vi "Fourier_Maple_Test.vi"() -> ()   [LabVIEW 2013]
uses:
  Hello Optotune Lens (30.06.2014)/Calibration.ctl
  <vilib>/Instr/_visa.llb/VISA Configure Serial Port (Instr).vi
panel:
  in  "f2k":dbl(slide)=114.95741056218058 min=80.0 max=200.0 scale=80.0..200.0
  in  "f1k":dbl(slide)=192.02725724020442 min=80.0 max=200.0 scale=80.0..200.0
  in  "Fourier/Abbildung":bool
  in  "f1i":dbl(slide)=80.0 min=80.0 max=200.0 step=5.0 scale=80.0..200.0
  in  "f2i":dbl(slide)=100.64735945485519 min=80.0 max=200.0 scale=80.0..200.0
  out "error out 2":errorcluster
  in  "error in (no error) 2":errorcluster
  in  "VISA resource name 2":string="COM14"
  out "I_min":dbl
  out "I_max":dbl
  in  "Calibration":T1={"Max Current A"=293.0, "Max Current B"=293.0, "UCL A"=300.0, "UCL B"=300.0, "LCL A"=0.0, "LCL B"=0.0} {"Max Current A" format="%#_g mA"; "Max Current B" format="%#_g mA"; "UCL A" format="%#_g mA"; "LCL A" format="%#_g mA"; "UCL B" format="%#_g mA"; "LCL B" format="%#_g mA"}
  out "ID":u16
  in  "Calibration 4":T1={"Max Current A"=293.0, "Max Current B"=293.0, "UCL A"=300.0, "UCL B"=300.0, "LCL A"=0.0, "LCL B"=0.0} {"Max Current A" format="%#_g mA"; "Max Current B" format="%#_g mA"; "UCL A" format="%#_g mA"; "LCL A" format="%#_g mA"; "UCL B" format="%#_g mA"; "LCL B" format="%#_g mA"}
  out "TA (°C) 2":dbl
  in  "Read Temperature 2":bool caption="Send Command"
  out "TA (°C)":dbl
  in  "Read Temperature":bool caption="Send Command"
  out "VISA resource name out 2":string="COM14"
  out "Calibration 3":T1={"Max Current A"=292.84, "Max Current B"=293.0, "UCL A"=292.76850585937495, "UCL B"=300.0, "LCL A"=4392.671494140624, "LCL B"=0.0} {"Max Current A" format="%#_g mA"; "Max Current B" format="%#_g mA"; "UCL A" format="%#_g mA"; "LCL A" format="%#_g mA"; "UCL B" format="%#_g mA"; "LCL B" format="%#_g mA"}
  out "OK 2":bool=TRUE
  out "Data 2":string
  out "Current Ch A (mA) 2":dbl=8.500677670604501
  out "Command to Port 2":string
  out "VISA resource name out":string="COM13"
  out "Calibration 2":T1={"Max Current A"=292.84, "Max Current B"=293.0, "UCL A"=292.76850585937495, "UCL B"=300.0, "LCL A"=4392.671494140624, "LCL B"=0.0} {"Max Current A" format="%#_g mA"; "Max Current B" format="%#_g mA"; "UCL A" format="%#_g mA"; "LCL A" format="%#_g mA"; "UCL B" format="%#_g mA"; "LCL B" format="%#_g mA"}
  out "OK":bool=TRUE
  out "Data":string
  out "Current Ch A (mA)":dbl=144.89333803039665
  out "Command to Port":string
  out "ID 2":u16
  out "error out":errorcluster={"status"=TRUE, "code"=-1073807360, "source"="Property Node (arg 1) in VISA Configure Serial Port (Instr).vi->Fourier_Maple_Test.vi"}
  in  "error in (no error)":errorcluster
  in  "VISA resource name":string="COM13"
  in  "Stop (F)":bool
  # "a_1 (Objekt->Linse vorderer Schraubanschluss) = 125mm\nd (Hinterer Schraubanschluss L1, Vorderer Schraubanschluss L2 = 151\na_2 (Hinterer Schraubanschluss L2, Sensor) =  13,28"
  # "d\tbeta_ges\ta_1\tpossensor\ta_2"
  # "95.45454545\t-0.691919192\t-150\t295.4545455\t50"
  # "82,67 114,54 192,92 102,67 f1i, f2i, f1k, f2k"
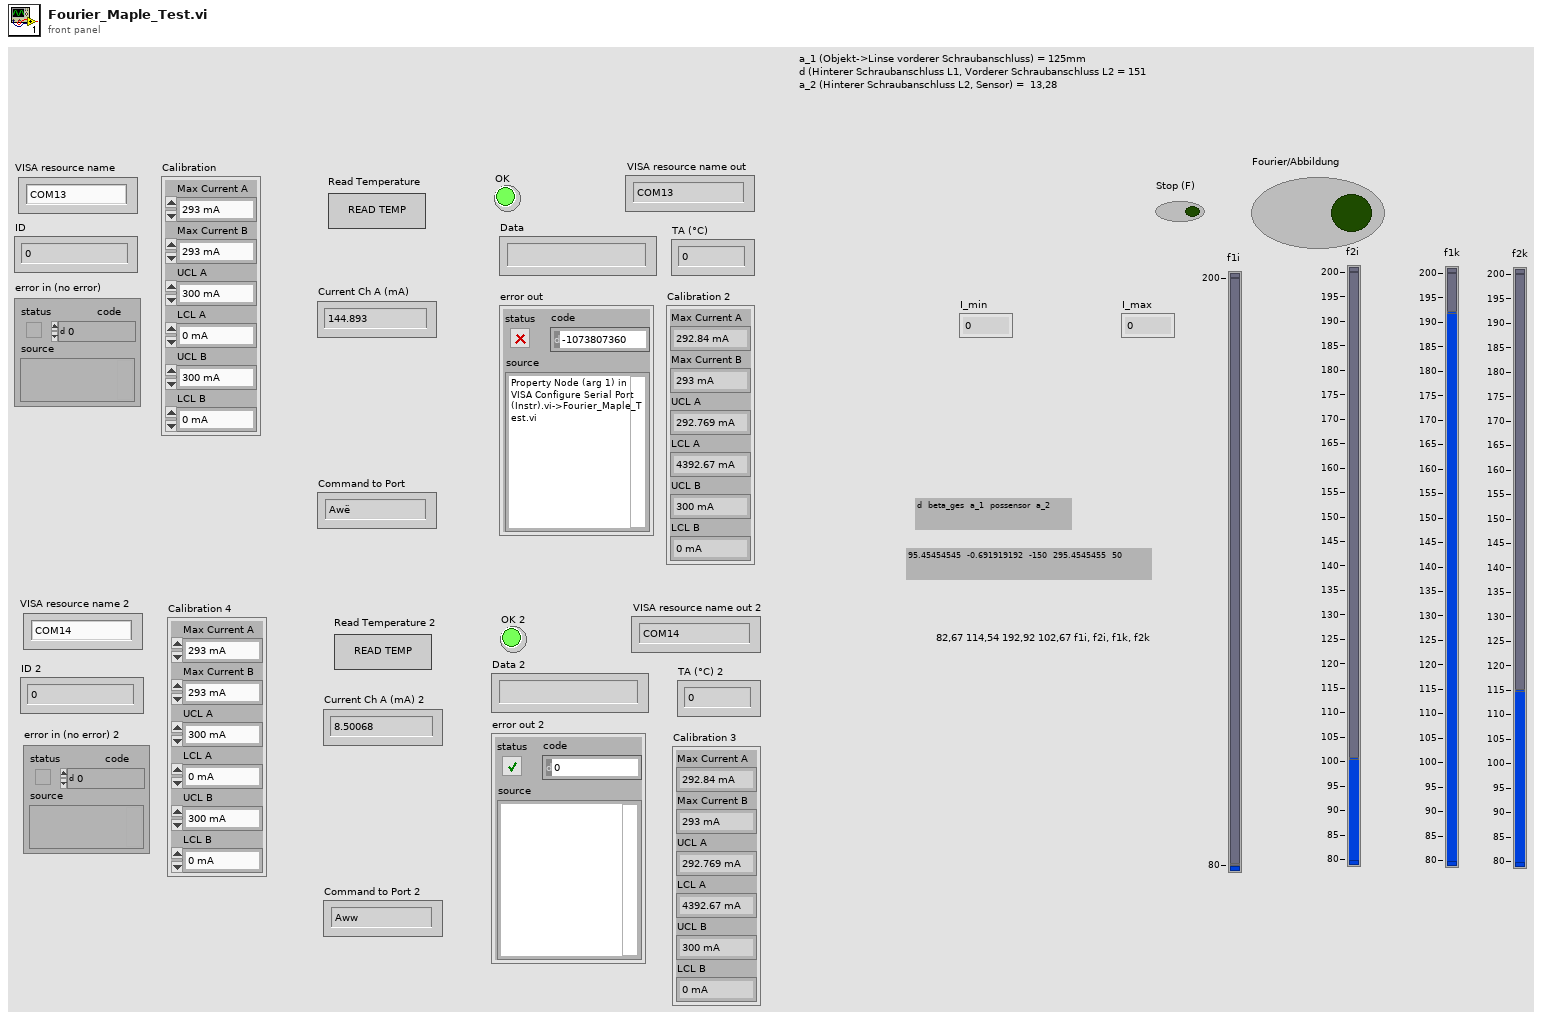
[diagram p1: front panel]
types:
  T1 = typedef "Calibration.ctl" = cluster{"Max Current A":dbl, "Max Current B":dbl, "UCL A":dbl, "UCL B":dbl, "LCL A":dbl, "LCL B":dbl}
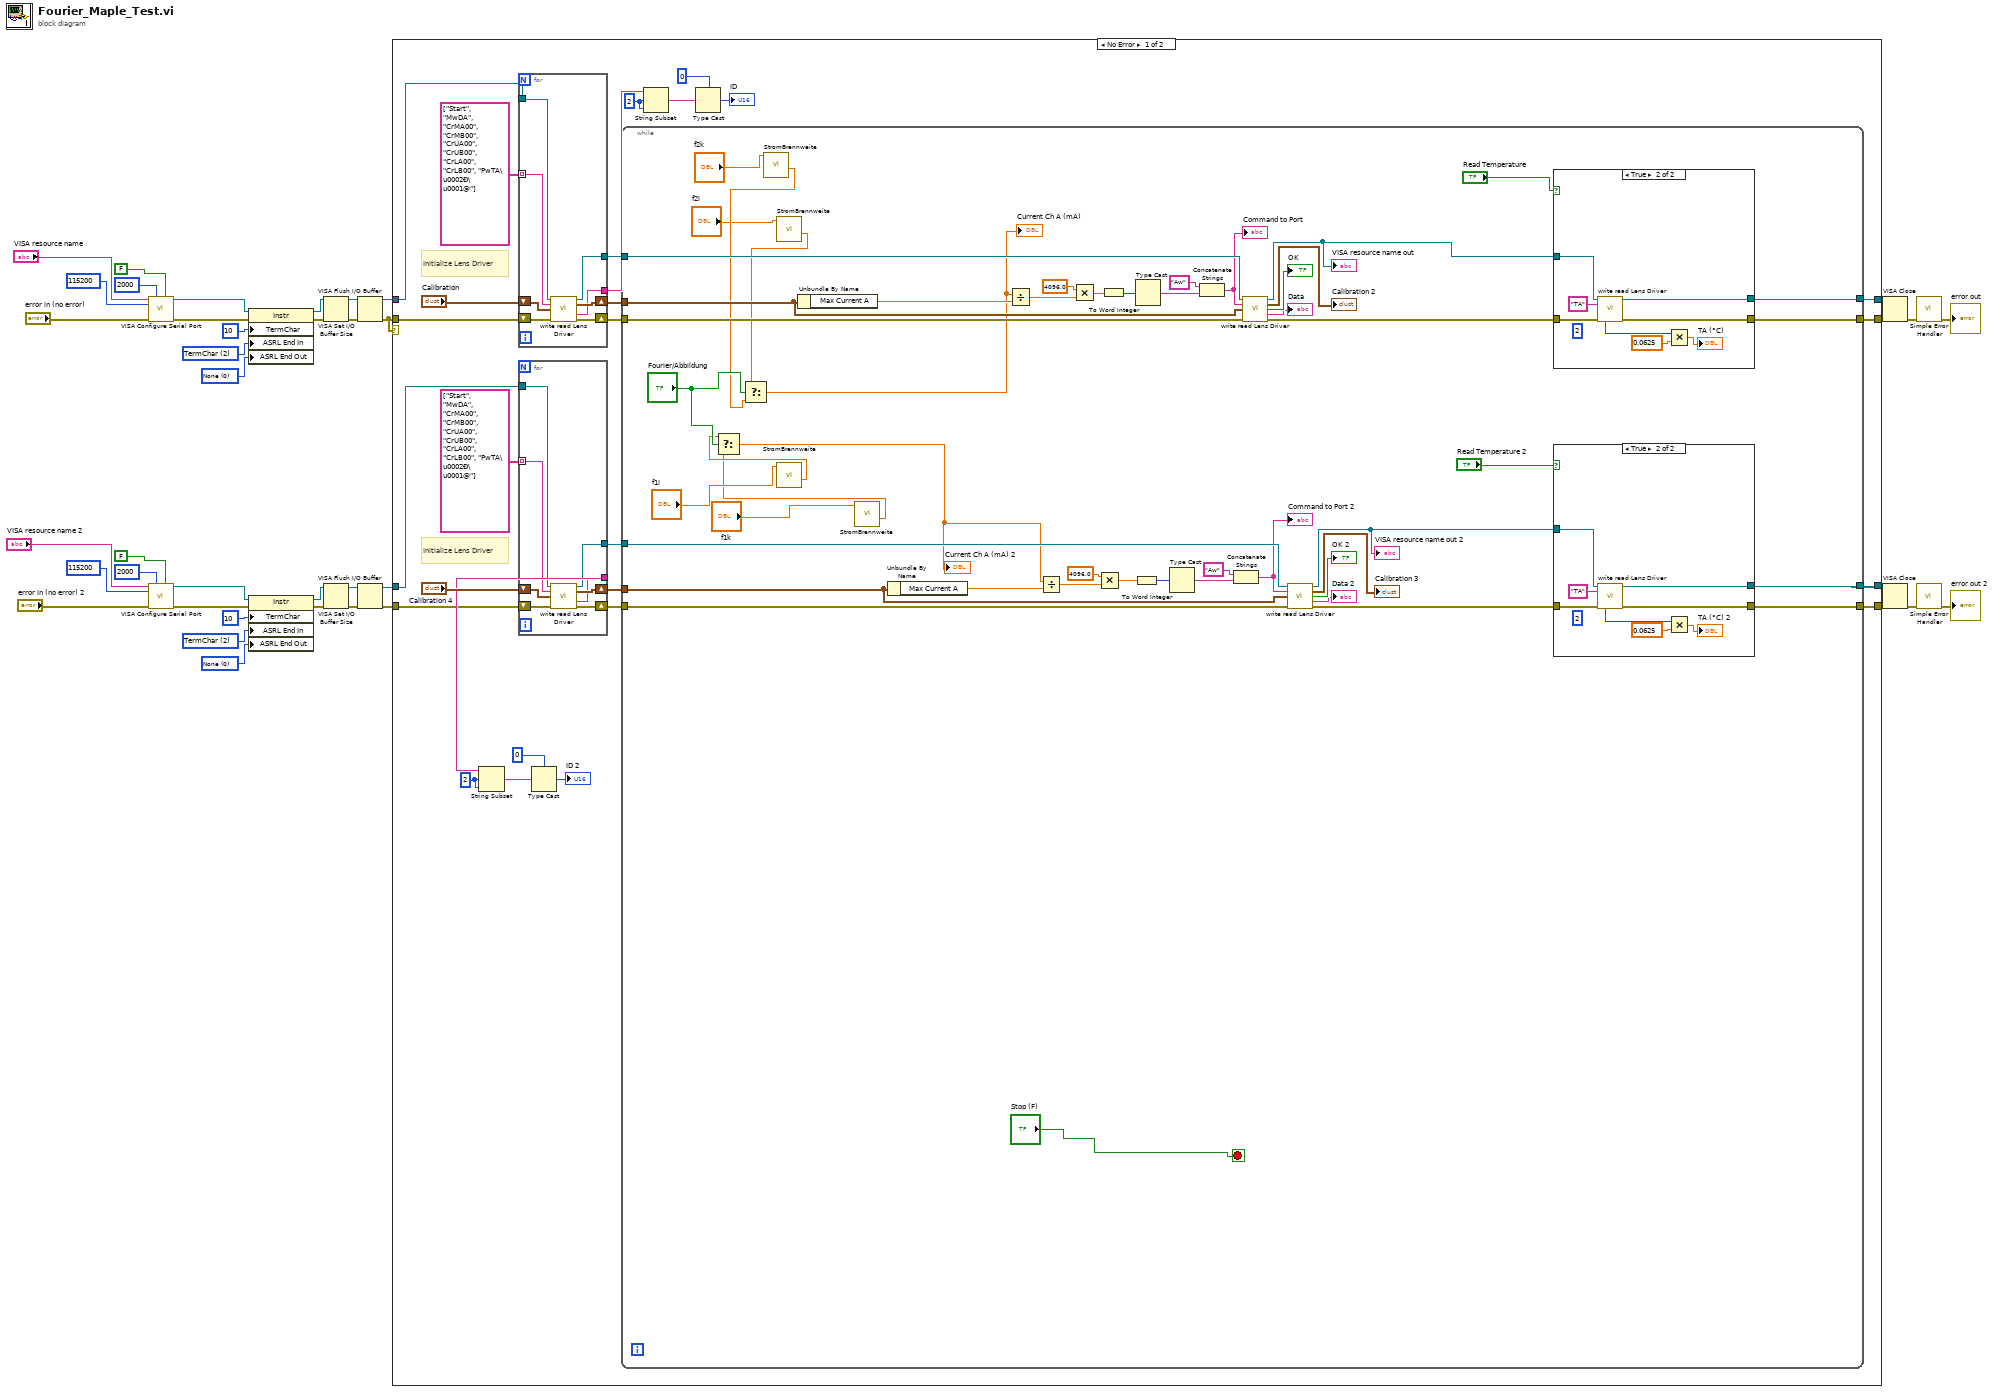
[diagram p0: block diagram]
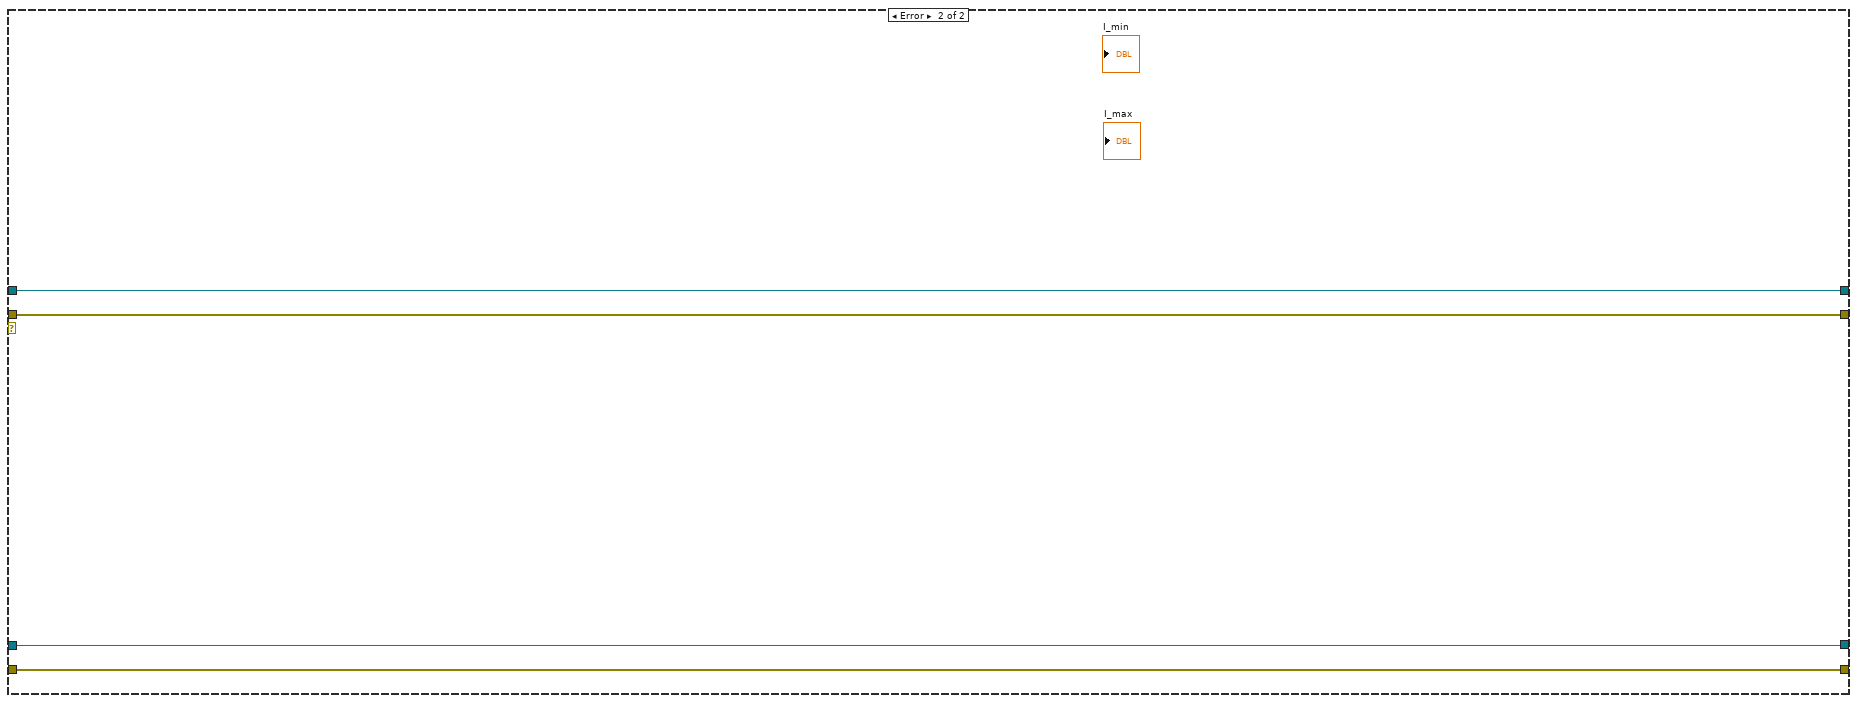
[diagram p4: hidden frame]
diagram:
  w11 = u16 0 items=["None", "Last Bit", "TermChar", "Break"] ("Serial Settings:End Mode for Writes")
  w12 = u16 2 items=["None", "Last Bit", "TermChar"] ("Serial Settings:End Mode for Reads")
  w31 = u16 0 items=["None", "Last Bit", "TermChar", "Break"] ("Serial Settings:End Mode for Writes")
  w32 = u16 2 items=["None", "Last Bit", "TermChar"] ("Serial Settings:End Mode for Reads")
  n1 = call-poly "VISA Configure Serial Port"("VISA resource name"="VISA resource name", "timeout (10sec)"=u32 2000, "Enable Termination\nChar (T)"=FALSE ("Enable Termination\nChar (T)"), "baud rate (9600)"=u32 115200, "error in (no error)"="error in (no error)") -> ("VISA resource name out"=w36:refnum<visa-resource-name>, "error out"=w34:errorcluster)  [unwired: 9 in]
  n2 = call-poly "VISA Configure Serial Port"("VISA resource name"="VISA resource name 2", "timeout (10sec)"=u32 2000, "Enable Termination\nChar (T)"=FALSE ("Enable Termination\nChar (T)"), "baud rate (9600)"=u32 115200, "error in (no error)"="error in (no error) 2") -> ("VISA resource name out"=w16:refnum<visa-resource-name>, "error out"=w14:errorcluster)  [unwired: 9 in]
  n3 = property class="Instr"(reference=w36, error in=w34, "TermChar"=u8 10 ("Message Based Settings:Termination Character"), "ASRL End In"=w32, "ASRL End Out"=w31) -> (reference out=w35:refnum<visa-resource-name>, error out=w33:errorcluster)
  n4 = property class="Instr"(reference=w16, error in=w14, "TermChar"=u8 10 ("Message Based Settings:Termination Character"), "ASRL End In"=w12, "ASRL End Out"=w11) -> (reference out=w15:refnum<visa-resource-name>, error out=w13:errorcluster)
  n5 = VISA Set I/O Buffer Size(VISA resource name=w35, error in (no error)=w33) -> (VISA resource name out=w28:refnum<visa-resource-name>, error out=w27:errorcluster)  [unwired: 2 in]
  n6 = VISA Set I/O Buffer Size(VISA resource name=w15, error in (no error)=w13) -> (VISA resource name out=w8:refnum<visa-resource-name>, error out=w7:errorcluster)  [unwired: 2 in]
  n7 = VISA Flush I/O Buffer(VISA resource name=w28, error in (no error)=w27) -> (VISA resource name out=w26:refnum<visa-resource-name>, error out=w21:errorcluster)  [unwired: 1 in]
  n8 = VISA Flush I/O Buffer(VISA resource name=w8, error in (no error)=w7) -> (VISA resource name out=w4:refnum<visa-resource-name>, error out=w3:errorcluster)  [unwired: 1 in]
  n9 = case shown="No Error" w21 {
    tunnel: w21 -> [w68 w157]
    tunnel: w26 -> [w67 w158]
    tunnel: [w66 w157] -> w24
    tunnel: [w65 w158] -> w22
    tunnel: w4 -> [w46 w156]
    tunnel: w3 -> [w45 w155]
    tunnel: [w42 w156] -> w2
    tunnel: [w41 w155] -> w1
    frame No Error {
      w53 = 2 ("length (rest)")
      w63 = 2 ("length (rest)")
      # "Initialize Lens Driver"
      # "Initialize Lens Driver"
      n10 = for {
        tunnel: w67 -> [w153]
        tunnel: [w150] -> w57
        tunnel: string[] ["Start", "MwDA", "CrMA00", "CrMB00", "CrUA00", "CrUB00", "CrLA00", "CrLB00", "PwTA\u0002Ð\u0001@"] -> [w148] mode=indexing
        tunnel: [w147] -> w56
        shift-right: [w151] -> w58
        shift-left: "Calibration" -> [w152]
        shift-right: [w149] -> w59
        shift-left: w68 -> [w154]
        n11 = call "write read Lens Driver.vi"("VISA resource name"=w153, "command"=w148, "Calibration"=w152, "error in (no error)"=w154) -> ("VISA resource name out"=w150:refnum<visa-resource-name>, "Calibration 2"=w151:T1, "Data"=w147:string, "error out"=w149:errorcluster)  [unwired: 4 in, 4 out]
      }
      n12 = for {
        tunnel: w46 -> [w145]
        tunnel: [w142] -> w48
        tunnel: string[] ["Start", "MwDA", "CrMA00", "CrMB00", "CrUA00", "CrUB00", "CrLA00", "CrLB00", "PwTA\u0002Ð\u0001@"] -> [w140] mode=indexing
        tunnel: [w139] -> w47
        shift-right: [w143] -> w49
        shift-left: "Calibration 4" -> [w144]
        shift-right: [w141] -> w50
        shift-left: w45 -> [w146]
        n13 = call "write read Lens Driver.vi"("VISA resource name"=w145, "command"=w140, "Calibration"=w144, "error in (no error)"=w146) -> ("VISA resource name out"=w142:refnum<visa-resource-name>, "Calibration 2"=w143:T1, "Data"=w139:string, "error out"=w141:errorcluster)  [unwired: 4 in, 4 out]
      }
      n14 = String Subset(string=w47, offset (0)=w53, length (rest)=w53) -> (substring=w51:string)
      n15 = Type Cast(type=u16 0 ("length (rest)"), x=w51) -> (*(type *) &x=→"ID 2":u16)
      n16 = while {
        tunnel: [w118] -> w66
        tunnel: [w117] -> w65
        tunnel: w59 -> [w116]
        tunnel: w58 -> [w115]
        tunnel: w57 -> [w114]
        tunnel: w50 -> [w113]
        tunnel: w49 -> [w112]
        tunnel: w48 -> [w111]
        tunnel: [w104] -> w42
        tunnel: [w103] -> w41
        stop <- "Stop (F)" stop-if-true
        n17 = call "StromBrennweite.vi"("f_var"="f2k") -> ("I_var_1"=w75:dbl)  [unwired: 8 in, 2 out]
        n18 = call "StromBrennweite.vi"("f_var"="f2i") -> ("I_var_1"=w73:dbl)  [unwired: 8 in, 2 out]
        n19 = Select(t=w73, s="Fourier/Abbildung", f=w75) -> (s? t:f=w80:dbl)
        "Current Ch A (mA)" <- w80
        n20 = call "StromBrennweite.vi"("f_var"="f1i") -> ("I_var_1"=w71:dbl)  [unwired: 8 in, 2 out]
        n21 = Unbundle By Name(w115) -> ("Max Current A"=w81:dbl)
        n22 = call "StromBrennweite.vi"("f_var"="f1k") -> ("I_var_1"=w69:dbl)  [unwired: 8 in, 2 out]
        n23 = Select(t=w71, s="Fourier/Abbildung", f=w69) -> (s? t:f=w78:dbl)
        "Current Ch A (mA) 2" <- w78
        n24 = Unbundle By Name(w112) -> ("Max Current A"=w92:dbl)
        n25 = Divide(x=w80, y=w81) -> (x/y=w88:dbl)
        n26 = Divide(x=w78, y=w92) -> (x/y=w99:dbl)
        n27 = Multiply(x=4096.0, y=w88) -> (x*y=w86:dbl)
        n28 = Multiply(x=4096.0, y=w99) -> (x*y=w97:dbl)
        n29 = To Word Integer(number=w86) -> (16bit integer=w85:i16)
        n30 = To Word Integer(number=w97) -> (16bit integer=w96:i16)
        n31 = Type Cast(x=w85) -> (*(type *) &x=w84:string)  [unwired: 1 in]
        n32 = Type Cast(x=w96) -> (*(type *) &x=w95:string)  [unwired: 1 in]
        n33 = Concatenate Strings("Aw", w84) -> (w82:string)
        "Command to Port" <- w82
        n34 = Concatenate Strings("Aw", w95) -> (w93:string)
        "Command to Port 2" <- w93
        n35 = call "write read Lens Driver.vi"("VISA resource name"=w114, "command"=w82, "Calibration"=w115, "error in (no error)"=w116) -> ("VISA resource name out"=w107:refnum<visa-resource-name>, "Calibration 2"=→"Calibration 2":T1, "OK"=→"OK":bool, "Data"=→"Data":string, "error out"=w106:errorcluster)  [unwired: 4 in, 3 out]
        "VISA resource name out" <- w107
        n36 = call "write read Lens Driver.vi"("VISA resource name"=w111, "command"=w93, "Calibration"=w112, "error in (no error)"=w113) -> ("VISA resource name out"=w110:refnum<visa-resource-name>, "Calibration 2"=→"Calibration 3":T1, "OK"=→"OK 2":bool, "Data"=→"Data 2":string, "error out"=w109:errorcluster)  [unwired: 4 in, 3 out]
        "VISA resource name out 2" <- w110
        n37 = case shown="True" "Read Temperature" {
          tunnel: [w120 w128] -> w117
          tunnel: [w119 w127] -> w118
          tunnel: w107 -> [w120 w126]
          tunnel: w106 -> [w119 w125]
          frame False {
          }
          frame True {
            (unwired) 2 ("length (rest)")
            n38 = call "write read Lens Driver.vi"("VISA resource name"=w126, "command"="TA", "error in (no error)"=w125) -> ("VISA resource name out"=w128:refnum<visa-resource-name>, "TA"=w122:u16, "error out"=w127:errorcluster)  [unwired: 5 in, 5 out]
            n39 = Multiply(x=w122, y=0.0625) -> (x*y=→"TA (°C)":dbl)
          }
        }
        n40 = case shown="True" "Read Temperature 2" {
          tunnel: [w130 w138] -> w104
          tunnel: [w129 w137] -> w103
          tunnel: w110 -> [w130 w136]
          tunnel: w109 -> [w129 w135]
          frame False {
          }
          frame True {
            (unwired) 2 ("length (rest)")
            n41 = call "write read Lens Driver.vi"("VISA resource name"=w136, "command"="TA", "error in (no error)"=w135) -> ("VISA resource name out"=w138:refnum<visa-resource-name>, "TA"=w132:u16, "error out"=w137:errorcluster)  [unwired: 5 in, 5 out]
            n42 = Multiply(x=w132, y=0.0625) -> (x*y=→"TA (°C) 2":dbl)
          }
        }
      }
      n43 = String Subset(string=w56, offset (0)=w63, length (rest)=w63) -> (substring=w61:string)
      n44 = Type Cast(type=u16 0 ("length (rest)"), x=w61) -> (*(type *) &x=→"ID":u16)
    }
    frame Error {
    }
  }
  n45 = VISA Close(VISA resource name=w22, error in (no error)=w24) -> (error out=w25:errorcluster)
  n46 = VISA Close(VISA resource name=w2, error in (no error)=w1) -> (error out=w6:errorcluster)
  n47 = call <vilib>:"Simple Error Handler.vi"("error in (no error)"=w25) -> ("error out"=→"error out":errorcluster)  [unwired: 4 in, 4 out]
  n48 = call <vilib>:"Simple Error Handler.vi"("error in (no error)"=w6) -> ("error out"=→"error out 2":errorcluster)  [unwired: 4 in, 4 out]
